vi "Load Electrical Network from Config.vi"(8 "error in":errorcluster, 11 "configuration file path":path) -> (0 "error out":errorcluster, 2 "NetworkData":T1[](array[typedef]), 3 "BusData":T2[](array[typedef]))   [LabVIEW 2018, in "Generic Optimization Actor.lvlib" / "Generic Optimization.lvclass"]
uses:
  Generic Optimization.lvclass
  Optimization Controls/Bus by ID.ctl
  <vilib>/ORNL/CSEISMIC DDS/CSEISMIC DDS Base/Data Types/Controls/DeviceID.ctl
  Optimization Controls/Electrical Network Optimization Data.ctl
  <vilib>/Utility/config.llb/Read Key (String).vi
  <vilib>/Utility/config.llb/Read Key (Double).vi
  <vilib>/Utility/config.llb/NI_LVConfig.lvlib
  <vilib>/ORNL/CSEISMIC DDS/CSEISMIC DDS Base/CSEISMIC DDS.lvclass
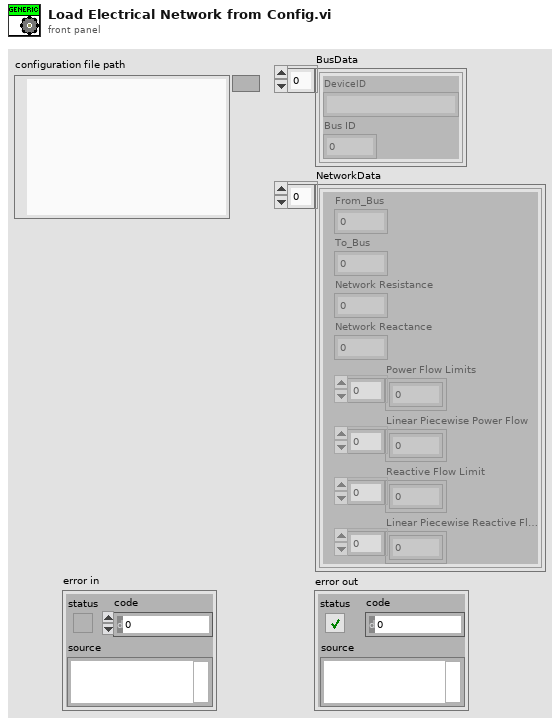
[diagram p1: front panel]
types:
  T1 = typedef "Generic Optimization Actor.lvlib/Generic Optimization.lvclass/Electrical Network Optimization Data.ctl" = cluster{"From_Bus":dbl, "To_Bus":dbl, "Network Resistance":dbl, "Network Reactance":dbl, "Power Flow Limits":dbl[], "Linear Piecewise Power Flow":dbl[], "Reactive Flow Limit":dbl[], "Linear Piecewise Reactive Flow":dbl[]}
  T2 = typedef "Generic Optimization Actor.lvlib/Generic Optimization.lvclass/Bus by ID.ctl" = cluster{"DeviceID":T3, "Bus ID":dbl}
  T3 = typedef "CSEISMIC DDS.lvlib/CSEISMIC DDS.lvclass/DeviceID.ctl" = string
  T4 = typedef "NI_LVConfig.lvlib/Config Data RefNum.ctl" = refnum<k1>
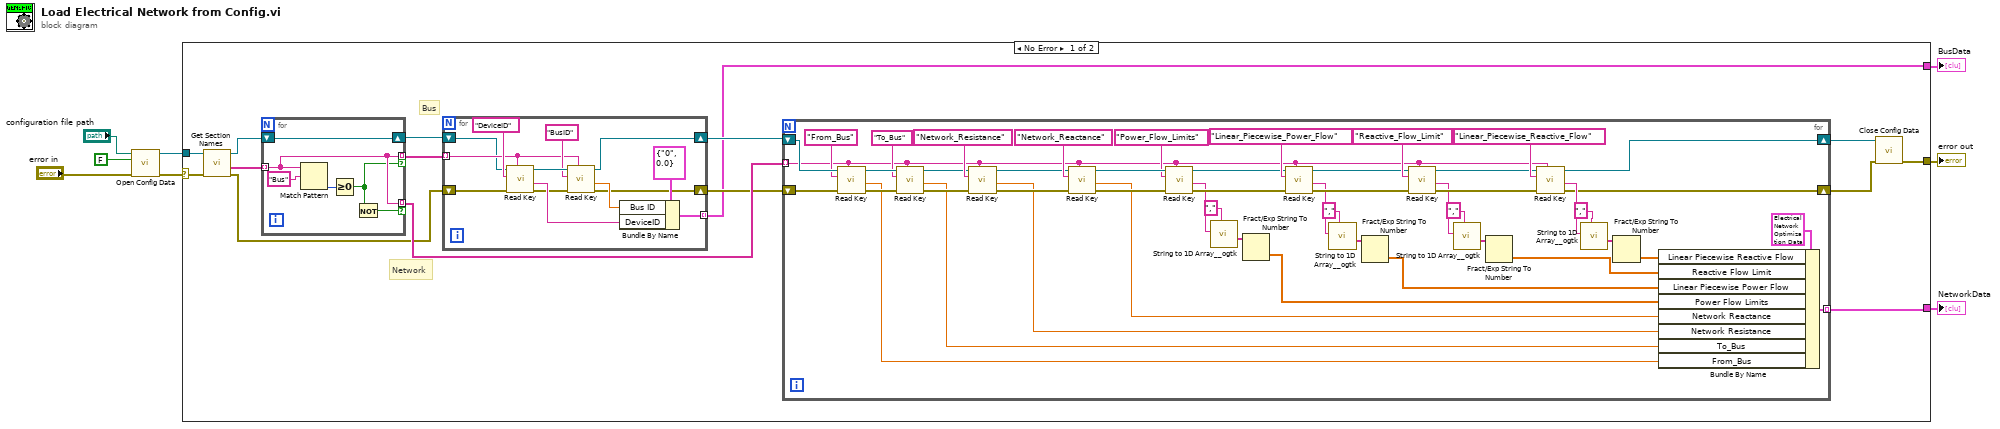
[diagram p0: block diagram]
diagram:
  n1 = call <vilib>:"Open Config Data.vi"("error in (no error)"="error in", "create file if necessary (T)"=FALSE, "configuration file path"="configuration file path") -> ("error out"=w6:errorcluster, "refnum"=w5:T4)  [unwired: 6 in, 1 out]
  n2 = case shown="No Error" w6 {
    selector: w6 -> [w22 w92]
    tunnel: [w9 w92] -> w1
    tunnel: w5 -> [w23 _]
    tunnel: [w13 _] -> w4
    tunnel: [w12 _] -> w3
    frame No Error {
      # "Network"
      # "Bus"
      n3 = call <vilib>:"Get Section Names.vi"("error in (no error)"=w22, "refnum"=w23) -> ("error out"=w15:errorcluster, "section names"=w21:string[], "refnum out"=w18:T4)  [unwired: 7 in]
      n4 = for {
        tunnel: w21 -> [w89] mode=indexing
        tunnel: [w89] -> w20 mode=indexing if=w87
        tunnel: [w89] -> w17 mode=indexing if=w88
        shift-right: [w86] -> w19
        shift-left: w18 -> [w86]
        n5 = Match Pattern(string=w89, regular expression="Bus") -> (offset past match=w90:i32)  [unwired: 1 in, 3 out]
        n6 = Greater Or Equal To 0?(x=w90) -> (x >= 0?=w87:bool)
        n7 = Not(x=w87) -> (.not. x?=w88:bool)
      }
      n8 = for {
        tunnel: w20 -> [w82] mode=indexing
        shift-right: [w80] -> w16
        shift-left: w19 -> [w81]
        tunnel: [w76] -> w13 mode=indexing
        shift-right: [w73] -> w14
        shift-left: w15 -> [w75]
        n9 = call-poly <vilib>:"Read Key.vi"("section"=w82, "error in (no error)"=w75, "key"="DeviceID", "refnum"=w81) -> ("error out"=w74:errorcluster, "value"=w78:string, "refnum out"=w84:T4)  [unwired: 4 in, 1 out]
        n10 = call-poly <vilib>:"Read Key.vi"("section"=w82, "error in (no error)"=w74, "key"="BusID", "refnum"=w84) -> ("error out"=w73:errorcluster, "value"=w79:dbl, "refnum out"=w80:T4)  [unwired: 4 in, 1 out]
        n11 = Bundle By Name(cluster=T2 {"DeviceID"="0", "Bus ID"=0.0} ("Bus by ID"), "Bus ID"=w79, "DeviceID"=w78) -> (w76:T2)
      }
      n12 = for {
        tunnel: w17 -> [w49] mode=indexing
        shift-right: [w34] -> w11
        shift-left: w16 -> [w72]
        shift-right: [w36] -> w10
        shift-left: w14 -> [w35]
        tunnel: [w24] -> w12 mode=indexing
        n13 = call-poly <vilib>:"Read Key.vi"("section"=w49, "error in (no error)"=w35, "key"="From_Bus", "refnum"=w72) -> ("error out"=w68:errorcluster, "value"=w25:dbl, "refnum out"=w70:T4)  [unwired: 4 in, 1 out]
        n14 = call-poly <vilib>:"Read Key.vi"("section"=w49, "error in (no error)"=w68, "key"="To_Bus", "refnum"=w70) -> ("error out"=w66:errorcluster, "value"=w26:dbl, "refnum out"=w65:T4)  [unwired: 4 in, 1 out]
        n15 = call-poly <vilib>:"Read Key.vi"("section"=w49, "error in (no error)"=w66, "key"="Network_Resistance", "refnum"=w65) -> ("error out"=w62:errorcluster, "value"=w27:dbl, "refnum out"=w63:T4)  [unwired: 4 in, 1 out]
        n16 = call-poly <vilib>:"Read Key.vi"("section"=w49, "error in (no error)"=w62, "key"="Network_Reactance", "refnum"=w63) -> ("error out"=w60:errorcluster, "value"=w28:dbl, "refnum out"=w61:T4)  [unwired: 4 in, 1 out]
        n17 = call-poly <vilib>:"Read Key.vi"("section"=w49, "error in (no error)"=w60, "key"="Power_Flow_Limits", "refnum"=w61) -> ("error out"=w52:errorcluster, "value"=w48:string, "refnum out"=w55:T4)  [unwired: 4 in, 1 out]
        n18 = call <userlib>:"String to 1D Array__ogtk.vi"("delimiter (Tab)"=",", "string"=w48) -> ("Array of Strings"=w46:string[])  [unwired: 9 in]
        n19 = Fract/Exp String To Number(string=w46) -> (number=w29:dbl[])  [unwired: 3 in, 1 out]
        n20 = call-poly <vilib>:"Read Key.vi"("section"=w49, "error in (no error)"=w52, "key"="Linear_Piecewise_Power_Flow", "refnum"=w55) -> ("error out"=w51:errorcluster, "value"=w39:string, "refnum out"=w54:T4)  [unwired: 4 in, 1 out]
        n21 = call <userlib>:"String to 1D Array__ogtk.vi"("delimiter (Tab)"=",", "string"=w39) -> ("Array of Strings"=w45:string[])  [unwired: 9 in]
        n22 = Fract/Exp String To Number(string=w45) -> (number=w30:dbl[])  [unwired: 3 in, 1 out]
        n23 = call-poly <vilib>:"Read Key.vi"("section"=w49, "error in (no error)"=w51, "key"="Reactive_Flow_Limit", "refnum"=w54) -> ("error out"=w50:errorcluster, "value"=w38:string, "refnum out"=w53:T4)  [unwired: 4 in, 1 out]
        n24 = call <userlib>:"String to 1D Array__ogtk.vi"("delimiter (Tab)"=",", "string"=w38) -> ("Array of Strings"=w44:string[])  [unwired: 9 in]
        n25 = Fract/Exp String To Number(string=w44) -> (number=w31:dbl[])  [unwired: 3 in, 1 out]
        n26 = call-poly <vilib>:"Read Key.vi"("section"=w49, "error in (no error)"=w50, "key"="Linear_Piecewise_Reactive_Flow", "refnum"=w53) -> ("error out"=w36:errorcluster, "value"=w37:string, "refnum out"=w34:T4)  [unwired: 4 in, 1 out]
        n27 = call <userlib>:"String to 1D Array__ogtk.vi"("delimiter (Tab)"=",", "string"=w37) -> ("Array of Strings"=w43:string[])  [unwired: 9 in]
        n28 = Fract/Exp String To Number(string=w43) -> (number=w32:dbl[])  [unwired: 3 in, 1 out]
        n29 = Bundle By Name(cluster=T1 {"From_Bus"=0.0, "To_Bus"=0.0, "Network Resistance"=0.0, "Network Reactance"=0.0, "Power Flow Limits"=[0.0, 0.0, 0.0], "Linear Piecewise Power Flow"=[0.0, 0.0, 0.0], "Reactive Flow Limit"=[0.0, 0.0, 0.0], "Linear Piecewise Reactive Flow"=[0.0, 0.0, 0.0]} ("Network Data"), "Linear Piecewise Reactive Flow"=w32, "Reactive Flow Limit"=w31, "Linear Piecewise Power Flow"=w30, "Power Flow Limits"=w29, "Network Reactance"=w28, "Network Resistance"=w27, "To_Bus"=w26, "From_Bus"=w25) -> (w24:T1)
      }
      n30 = call <vilib>:"Close Config Data.vi"("error in (no error)"=w10, "refnum"=w11) -> ("error out"=w9:errorcluster)  [unwired: 8 in, 1 out]
    }
    frame Error {
    }
  }
  "BusData" <- w4
  "NetworkData" <- w3
  "error out" <- w1
